vi "UpdateStreamingFilterIDs.vi"(8 "error in (no error)":errorcluster, 10 "IDs":u32[](array[numeric]), 11 "Ref":T1) -> (0 "error out":errorcluster, 3 "Ref":T1)   [LabVIEW 2019, in "Diagnostics Host Automation API.lvlib"]
uses:
  Diagnostics Host Automation API.lvlib
  Addon/Addon Shared/Types/HostAutomation.Ref.ctl
  <vilib>/NI/STM/TCP/TCP Connection Info.ctl
  <vilib>/NI/STM/SubVIs/MetaDataElement.ctl
  Addon/Addon Shared/Types/DTC.Codes.ctl
  <vilib>/NI/NI VeriStand Addon Network Comm/Shared/NI VeriStand Addon Network Comm Shared.lvlib
  <vilib>/NI/STM/NI STM.lvlib
  Addon/Addon Shared/Diagnostics Addon Shared.lvlib
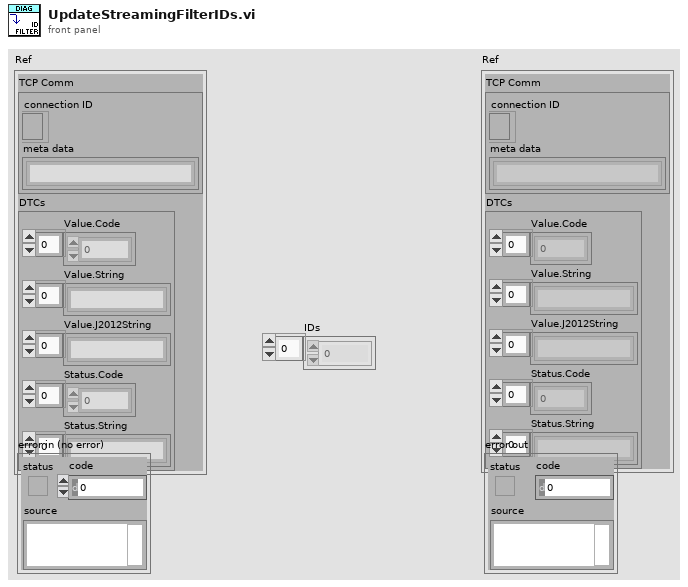
[diagram p1: front panel]
types:
  T1 = typedef "Diagnostics Addon Shared.lvlib/HostAutomation.Ref.ctl" = cluster{"TCP Comm":T2, "DTCs":T4}
  T2 = typedef "NI STM.lvlib/TCP Connection Info.ctl" = cluster{"connection ID":refnum<k5>, "meta data":T3[]}
  T3 = typedef "NI STM.lvlib/MetaDataElement.ctl" = string
  T4 = typedef "Diagnostics Addon Shared.lvlib/DTC.Codes.ctl" = cluster{"Value.Code":dbl[], "Value.String":string[], "Value.J2012String":string[], "Status.Code":dbl[], "Status.String":string[]}
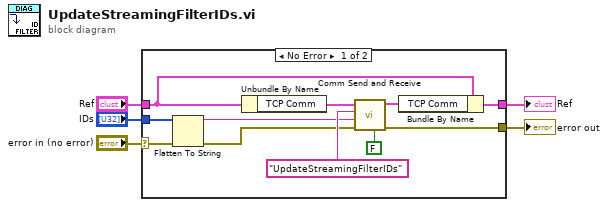
[diagram p0: block diagram]
diagram:
  n1 = case shown="No Error" "error in (no error)" {
    selector: "error in (no error)" -> [w9 w18]
    tunnel: "Ref" -> [w12 w17]
    tunnel: [w10 w17] -> w4
    tunnel: [w16 w18] -> w3
    tunnel: "IDs" -> [w7 _]
    frame No Error {
      n2 = Flatten To String(anything=w7, error in (no error)=w9) -> (data string=w6:string, error out=w8:errorcluster)  [unwired: 2 in, 1 out]
      n3 = Unbundle By Name(w12) -> ("TCP Comm"=w13:T2)
      n4 = call <vilib>:"Comm Send and Receive.vi"("Resp Required?"=FALSE, "error in (no error)"=w8, "Data"=w6, "Name"="UpdateStreamingFilterIDs", "connection info"=w13) -> ("error out"=w16:errorcluster, "connection info"=w11:T2)  [unwired: 3 in, 2 out]
      n5 = Bundle By Name(cluster=w12, "TCP Comm"=w11) -> (w10:T1)
    }
    frame Error {
    }
  }
  "Ref" <- w4
  "error out" <- w3
